vi "newid.vi"(11 "client handle":T1) -> (3 "client handle out":T1)   [LabVIEW 2012]
uses:
  Key-Value Pair.ctl
  <vilib>/httpClient/ClientHandle.ctl
  <vilib>/httpClient/LabVIEWHTTPClient.lvlib
panel:
  out "Parsed Headers":T2[](array[typedef])
  out "body":string
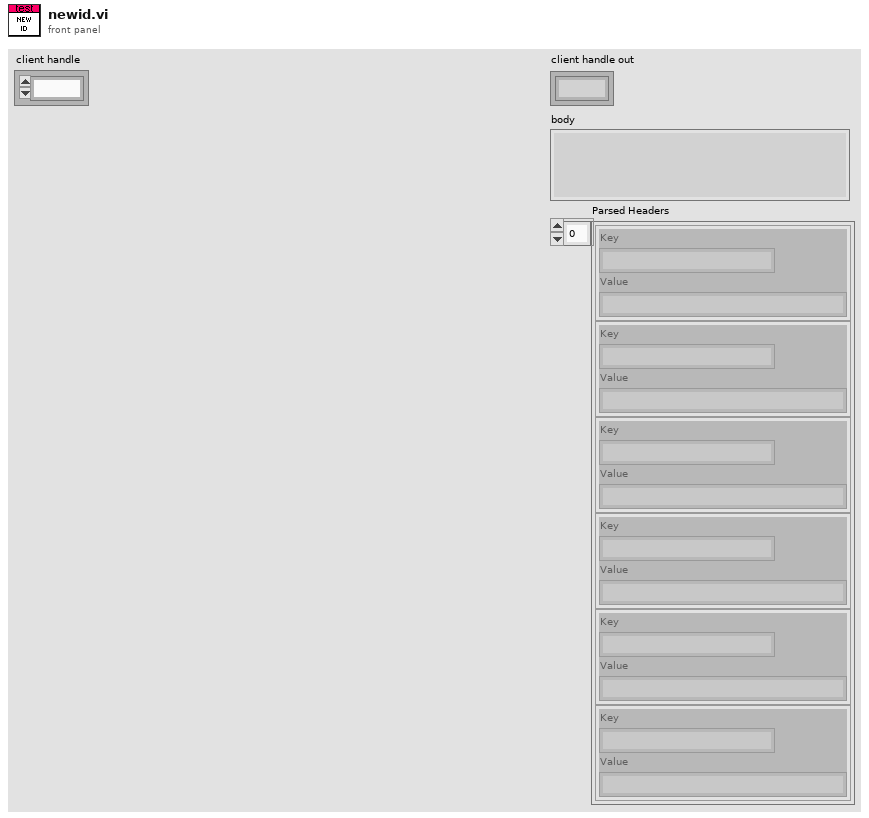
[diagram p1: front panel]
types:
  T1 = typedef "LabVIEWHTTPClient.lvlib/ClientHandle.ctl" = refnum<k1>
  T2 = typedef "Key-Value Pair.ctl" = cluster{"Key":string, "Value":string}
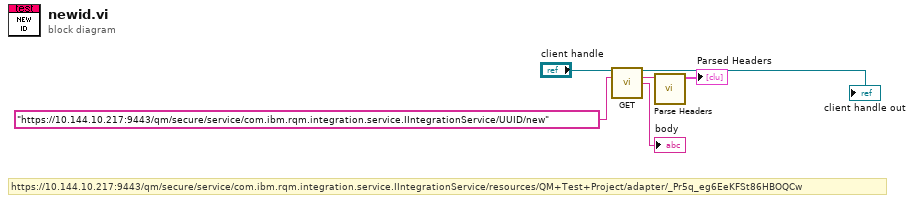
[diagram p0: block diagram]
diagram:
  # "https://10.144.10.217:9443/qm/secure/service/com.ibm.rqm.integration.service.IIntegrationService/resources/QM+Test+Project/adapter/_Pr5q_eg6EeKFSt86HBOQCw"
  n1 = call <vilib>:"GET.vi"("client handle"="client handle", "url"="https://10.144.10.217:9443/qm/secure/service/com.ibm.rqm.integration.service.IIntegrationService/UUID/new") -> ("client handle out"=→"client handle out":T1, "headers"=w5:string, "body"=→"body":string)  [unwired: 10 in, 1 out]
  n2 = call "Parse Headers.vi"("Raw Header"=w5) -> ("Parsed Headers"=→"Parsed Headers":T2[])  [unwired: 9 in, 1 out]
